vi "Handle Topology Change.vi"(8 "error in (no error)":errorcluster, 10 "Topology":string, 11 "SLSC Switch Custom Device Ref in":T1 format="%.0x") -> (0 "error out":errorcluster, 3 "SLSC Switch Custom Device Ref out":T1 format="%.0x")   [LabVIEW 2017, in "SLSC Switch System Explorer.lvlib"]
uses:
  SLSC Switch System Explorer.lvlib
  <vilib>/NI Veristand/Custom Device API/Custom Device Item Ref.ctl
  Scripting/SLSC Switch Scripting.lvlib
  <vilib>/NI Veristand/Custom Device API/Custom Device API.lvlib
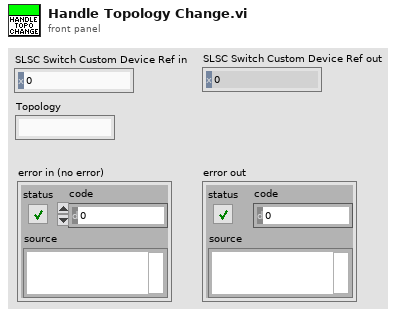
[diagram p1: front panel]
types:
  T1 = typedef "Custom Device API.lvlib/Custom Device Item Ref.ctl" = u64
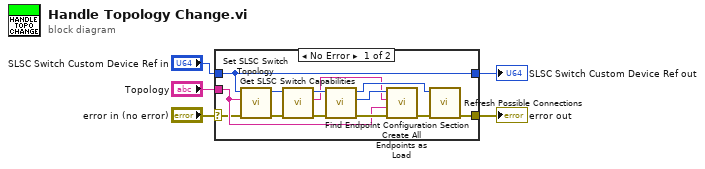
[diagram p0: block diagram]
diagram:
  n1 = case shown="No Error" "error in (no error)" {
    selector: "error in (no error)" -> [w7 w20]
    tunnel: [w6 w19] -> w5
    tunnel: "SLSC Switch Custom Device Ref in" -> [w6 w19]
    tunnel: "Topology" -> [w11 _]
    tunnel: [w8 w20] -> w2
    frame No Error {
      n2 = call "Set SLSC Switch Topology.vi"("error in (no error)"=w7, "Topology"=w11, "SLSC Switch Custom Device Ref in"=w6) -> ("error out"=w10:errorcluster, "SLSC Switch Custom Device Ref out"=w18:T1)  [unwired: 7 in]
      n3 = call "Get SLSC Switch Capabilities.vi"("error in (no error)"=w10, "SLSC Switch Custom Device Ref in"=w18) -> ("error out"=w14:errorcluster, "Capabilities"=w12:string, "SLSC Switch Custom Device Ref out"=w13:T1)  [unwired: 7 in]
      n4 = call "Find Endpoint Configuration Section.vi"("error in (no error)"=w14, "SLSC Switch Custom Device Ref in"=w13) -> ("error out"=w15:errorcluster, "Endpoint Config Section Ref"=w16:T1, "SLSC Switch Custom Device Ref out"=w17:T1)  [unwired: 7 in]
      n5 = call "Create All Endpoints as Load.vi"("error in (no error)"=w15, "topology"=w11, "switches json"=w12, "Endpoint Config Section Ref"=w16) -> ("error out"=w9:errorcluster)  [unwired: 6 in, 1 out]
      n6 = call "Refresh Possible Connections.vi"("error in (no error)"=w9, "SLSC Switch Custom Device Ref in"=w17) -> ("error out"=w8:errorcluster)  [unwired: 8 in, 1 out]
    }
    frame Error {
    }
  }
  "SLSC Switch Custom Device Ref out" <- w5
  "error out" <- w2
